vi "DefineFunctionStart.vi"(7 "Function name":string="test()", 8 "return":string, 9 "Function":T1, 11 "Data In":T1) -> (3 "Data Out":T1={"Port"="", "All Code"="Hi"})   [LabVIEW 2016]
uses:
  uPythonX/PythonData.ctl
  uPythonX/uPythonX.xctl
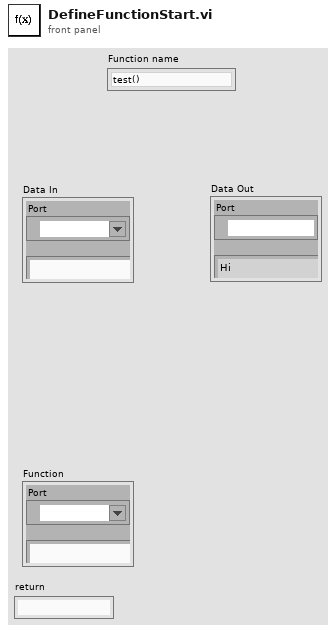
[diagram p1: front panel]
types:
  T1 = typedef "uPythonX.xctl/PythonData.ctl" = cluster{"Port":refnum<visa-resource-name>, "All Code":string}
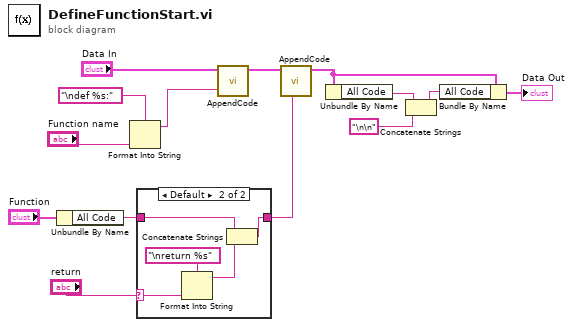
[diagram p0: block diagram]
diagram:
  n1 = Unbundle By Name("Function") -> ("All Code"=w3:string)
  n2 = Format Into String(format string="\ndef %s:", "Function name") -> (resulting string=w11:string)  [unwired: 2 in, 1 out]
  n3 = case shown="Default" "return" {
    selector: "return" -> [_ w17]
    tunnel: w3 -> [w15 w16]
    tunnel: [w15 w20] -> w2
    frame "" {
    }
    frame Default {
      n4 = Format Into String(format string="\nreturn %s", w17) -> (resulting string=w18:string)  [unwired: 2 in, 1 out]
      n5 = Concatenate Strings(w16, w18) -> (w20:string)
    }
  }
  n6 = call "AppendCode.vi"("New Code"=w11, "Data In"="Data In") -> ("Data Out"=w6:T1)  [unwired: 9 in]
  n7 = call "AppendCode.vi"("New Code"=w2, "Data In"=w6) -> ("Data Out"=w5:T1)  [unwired: 9 in]
  n8 = Unbundle By Name(w5) -> ("All Code"=w8:string)
  n9 = Concatenate Strings(w8, "\n\n" ("New Code")) -> (w10:string)
  n10 = Bundle By Name(cluster=w5, "All Code"=w10) -> (→"Data Out":T1)
